vi "GDX_TwoSensors.vi"() -> ()   [LabVIEW 2019]
panel:
  out "XY Graph 2":cluster{dbl[], dbl[]}[](graph)
  out "XY Graph 1":cluster{dbl[], dbl[]}[](graph)
  in  "stop":bool
  out "error out":errorcluster
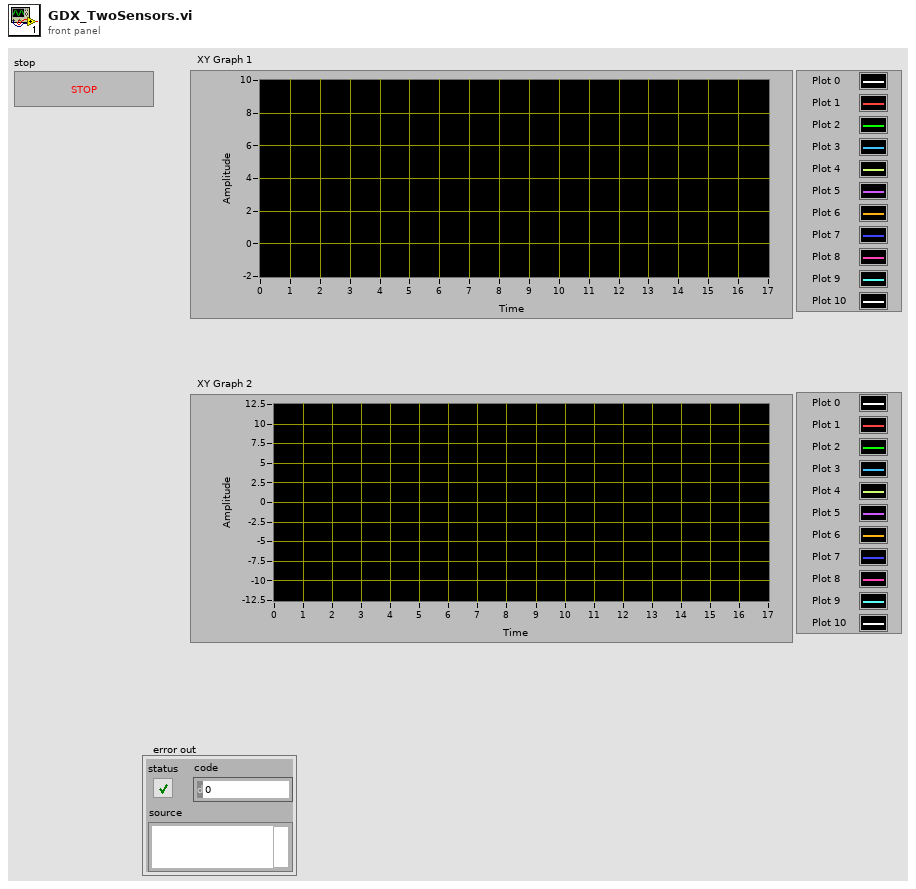
[diagram p1: front panel]
types:
  T1 = enum16{"Open from Dialog Popup", "Open all Available Devices", "Input Device Names"}
  T2 = enum16{"Activate from Dialog Popup", "Activate All Channels", "Input On/Off Array", "Input Channel  Mask", "Burn Sensor Default Channels"}
  T3 = enum16{"Set Rate from Dialog Popup", "Default 1 Sample/Sec", "Input Sample Rate"}
  T4 = typedef "D2PIO_D2PIOCluster.ctl" = cluster{"Library Handle":i64, "Device List Handle":i64, "BT Device Handles":i64[], "USB Device Handles":i64[], "BT+USB Device Handles":i64[], "Measurement Tick":dbl[], "Ch Availability Mask":u32[]}
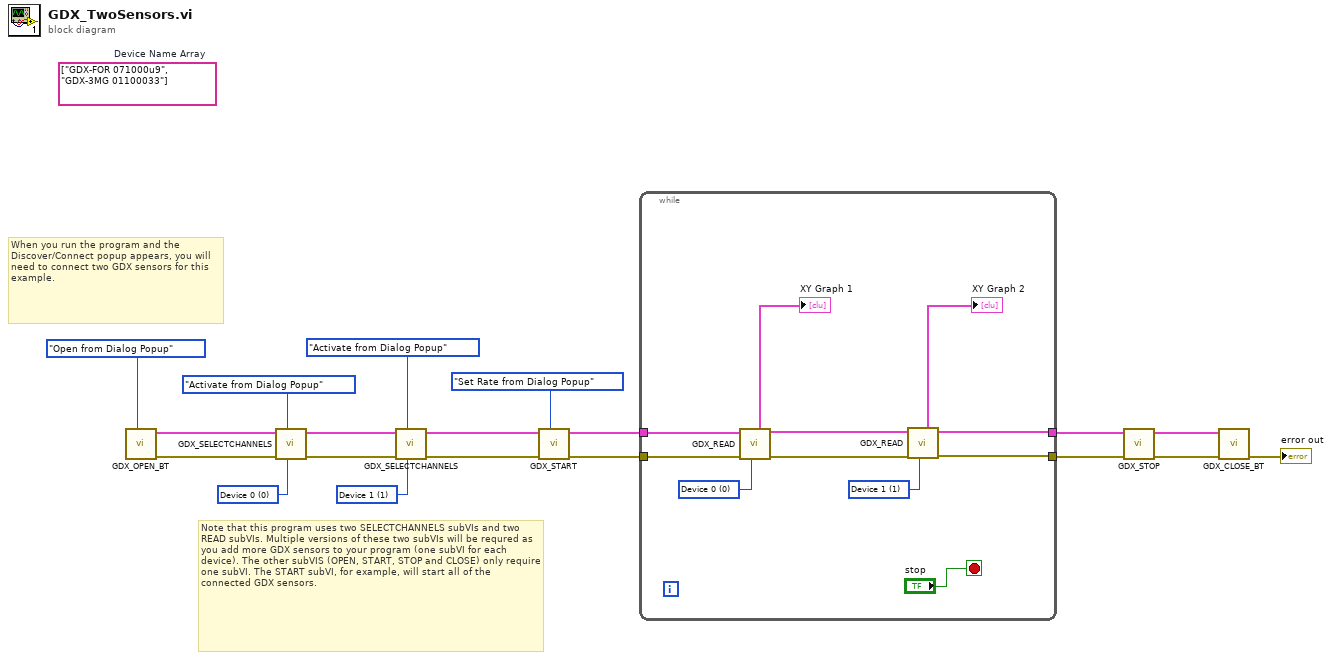
[diagram p0: block diagram]
diagram:
  w5 = 1 items=["Device 0", "Device 1", "Device 2", "Device 3", "Device 4", "Device 5", "Device 6", "Device 7", "Device 8", "Device 9", "Device 10", "Device 11"] ("Device Index")
  w6 = 0 items=["Device 0", "Device 1", "Device 2", "Device 3", "Device 4", "Device 5", "Device 6", "Device 7", "Device 8", "Device 9", "Device 10", "Device 11"] ("Device Index")
  (unwired) string[] ["GDX-FOR 071000u9", "GDX-3MG 01100033"]  # Device Name Array
  # "When you run the program and the Discover/Connect popup appears, you will need to connect two GDX sensors for this example."
  # "Note that this program uses two SELECTCHANNELS subVIs and two READ subVIs. Multiple versions of these two subVIs will be requred as you add more GDX sensors to your program (one subVI for each device). The other subVIS (OPEN, START, STOP and CLOSE) only require one subVI. The START subVI, for example, will start all of the connected GDX sensors."
  n1 = call <vilib>:"GDX_OPEN_BT.vi"("Enum"=T1."Open from Dialog Popup") -> ("error out"=w12:errorcluster, "D2PIO Cluster Out"=w13:T4)  [unwired: 9 in]
  n2 = call <vilib>:"GDX_SELECTCHANNELS.vi"("Device Index"=w6, "Enum"=T2."Activate from Dialog Popup", "error in (no error)"=w12, "D2PIO Cluster In"=w13) -> ("error out"=w9:errorcluster, "D2PIO Cluster Out"=w10:T4)  [unwired: 6 in]
  n3 = call <vilib>:"GDX_SELECTCHANNELS.vi"("Device Index"=w5, "Enum"=T2."Activate from Dialog Popup", "error in (no error)"=w9, "D2PIO Cluster In"=w10) -> ("error out"=w7:errorcluster, "D2PIO Cluster Out"=w8:T4)  [unwired: 6 in]
  n4 = call <vilib>:"GDX_START.vi"("Enum"=T3."Set Rate from Dialog Popup", "error in (no error)"=w7, "D2PIO Cluster In"=w8) -> ("error out"=w19:errorcluster, "D2PIO Cluster Out"=w18:T4)  [unwired: 5 in, 2 out]
  n5 = while {
    tunnel: w19 -> [w30]
    tunnel: w18 -> [w28]
    tunnel: [w25] -> w17
    tunnel: [w24] -> w11
    stop <- "stop" stop-if-true
    w20 = 1 items=["Device 0", "Device 1", "Device 2", "Device 3", "Device 4", "Device 5", "Device 6", "Device 7", "Device 8", "Device 9", "Device 10", "Device 11"] ("Device Index")
    w21 = 0 items=["Device 0", "Device 1", "Device 2", "Device 3", "Device 4", "Device 5", "Device 6", "Device 7", "Device 8", "Device 9", "Device 10", "Device 11"] ("Device Index")
    n6 = call <vilib>:"GDX_READ.vi"("Device Index"=w21, "error in (no error)"=w30, "D2PIO Cluster In"=w28) -> ("error out"=w27:errorcluster, "D2PIO Cluster Out"=w26:T4, "XY Graph Data"=→"XY Graph 1":cluster{dbl[], dbl[]}[])  [unwired: 3 in, 3 out]
    n7 = call <vilib>:"GDX_READ.vi"("Device Index"=w20, "error in (no error)"=w27, "D2PIO Cluster In"=w26) -> ("error out"=w24:errorcluster, "D2PIO Cluster Out"=w25:T4, "XY Graph Data"=→"XY Graph 2":cluster{dbl[], dbl[]}[])  [unwired: 3 in, 3 out]
  }
  n8 = call <vilib>:"GDX_STOP.vi"("error in (no error)"=w11, "D2PIO Cluster In"=w17) -> ("error out"=w15:errorcluster, "D2PIO Cluster Out"=w16:T4)  [unwired: 8 in]
  n9 = call <vilib>:"GDX_CLOSE_BT.vi"("error in (no error)"=w15, "D2PIO Cluster In"=w16) -> ("error out"=→"error out":errorcluster)  [unwired: 8 in, 1 out]
